vi "Pockels-Calc sequence length in ms.vi"(11 "Pockels modulation sequence in":dbl[](array[numeric])) -> (1 "Sequence length (points)":i32, 3 "Sequence length (ms)":dbl, 4 "Sampling period (us)":dbl=1e-06)   [LabVIEW 2020]
uses:
  Global Variables/General Globals.vi
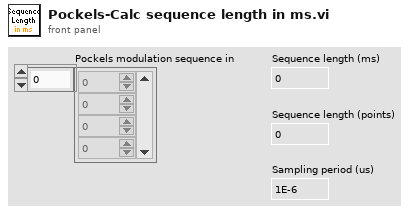
[diagram p1: front panel]
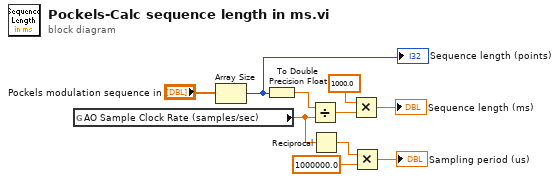
[diagram p0: block diagram]
diagram:
  n1 = global read "General Globals.vi" "AO Sample Clock Rate (samples/sec)"() -> (w4:dbl)
  n2 = Array Size(array="Pockels modulation sequence in") -> (size(s)=w5:i32)
  "Sequence length (points)" <- w5
  n3 = To Double Precision Float(number=w5) -> (double precision float=w9:dbl)
  n4 = Divide(x=w9, y=w4) -> (x/y=w7:dbl)
  n5 = Reciprocal(x=w4) -> (1/x=w2:dbl)
  n6 = Multiply(x=1000.0, y=w7) -> (x*y=→"Sequence length (ms)":dbl)
  n7 = Multiply(x=w2, y=1000000.0) -> (x*y=→"Sampling period (us)":dbl)
